vi "DS_WLs.vi"(6 "Wavelengths":dbl[](array[numeric]), 7 "Pixel numbers":i32[](array[numeric]), 9 "Pixels":i32) -> (1 "Pixels":i32[](array[numeric]), 2 "DSd WLs":dbl[](array[numeric]))   [LabVIEW 2019]
uses:
  <vilib>/gmath/NI_Gmath.lvlib
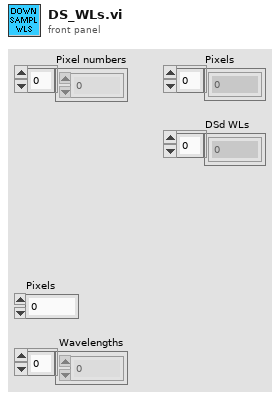
[diagram p1: front panel]
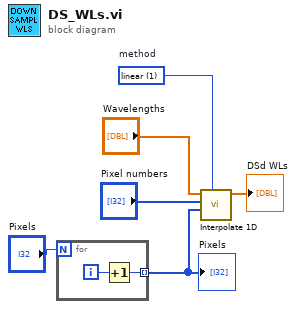
[diagram p0: block diagram]
diagram:
  w4 = 1 items=["nearest", "linear", "spline", "cubic Hermite", "Lagrange"]  # method
  n1 = for {
    N: "Pixels" -> [_]
    tunnel: [w7] -> w5 mode=indexing
    i -> [w8]
    n2 = Increment(x=w8) -> (x+1=w7:i32)
  }
  "Pixels" <- w5
  n3 = call <vilib>:"Interpolate 1D.vi"("method"=w4, "xi"=w5, "X"="Pixel numbers", "Y"="Wavelengths") -> ("yi"=→"DSd WLs":dbl[])  [unwired: 5 in, 2 out]
